vi "UpdateFlagState.vi"(7 "LabVIEW Web Service Request":refnum<class "Web Request.lvclass">, 9 "Room":i32, 10 "FlagState":u32) -> (2 "FlagOut":string)   [LabVIEW 2015]
uses:
  <vilib>/wsapi/Web Request.lvclass
  TypeDef/ActionEnum.ctl
panel:
  # "Use the Web Service Request input terminal to call the VIs on the Web Services palette. Do not remove it from the connector pane unless you don't need access to the palette."
  # "Each additional control wired to the connector pane will be available as an input in the URL. To include an indicator in terminal-mode output (the default setting), it must also be wired to the connector pane."
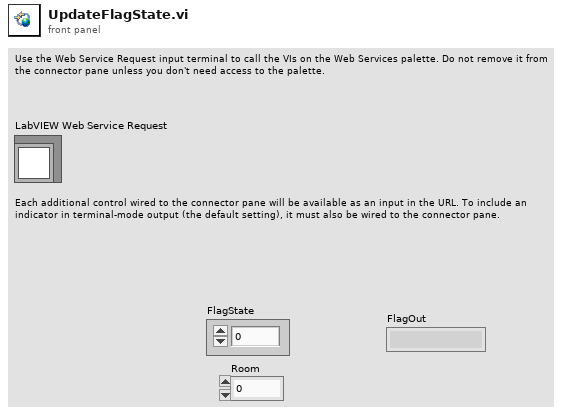
[diagram p1: front panel]
types:
  T1 = typedef "ActionEnum.ctl" = enum16{"Init", "Add Room", "Remove Room", "Read Room", "Read Flag", "Read Flag State", "Write Flag State", "Read Flag Color", "Write Flag Color", "Read Bed Vacant", "Write Bed Vacant", "Read Personnel", "Add Personnel", "Remove Personnel", "Read Requests", "Add Request", "Remove Request", "Read Beacon ID", "Write Beacon ID", "Write Bed URL", "Read Bed URL"}
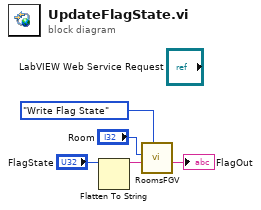
[diagram p0: block diagram]
diagram:
  n1 = Flatten To String(anything="FlagState") -> (data string=w2:string)  [unwired: 3 in, 2 out]
  n2 = call "RoomsFGV.vi"("Actions"=ActionEnum."Write Flag State", "Data In"=w2, "Room"="Room") -> ("Data Out"=→"FlagOut":string)  [unwired: 7 in, 1 out]
